vi "main.vi"() -> ()   [LabVIEW 2024]
uses:
  Controller/Controller/Controller.lvclass
  Applications/National Instruments/LabVIEW 2024 64-bit/vi.lib/ActorFramework/Actor/Actor.lvclass
  <vilib>/ActorFramework/Message Enqueuer/Message Enqueuer.lvclass/Message Enqueuer.ctl
  <vilib>/ActorFramework/Message Enqueuer/Enqueue.vi
  Controller/Controller Messages/Reset Contestant Lights Msg/Reset Contestant Lights Msg.lvclass
  Applications/National Instruments/LabVIEW 2024 64-bit/vi.lib/ActorFramework/Message/Message.lvclass
  <vilib>/ActorFramework/Stop Msg/Stop Msg.lvclass
  Controller/Controller Messages/Welcome Animation Msg/Welcome Animation Msg.lvclass
  <vilib>/ActorFramework/Message Priority Queue/Priority Enqueue.vi
  <vilib>/ActorFramework/Actor/Actor.lvclass
panel:
  in  "Hype":bool
  in  "Stop Button":bool
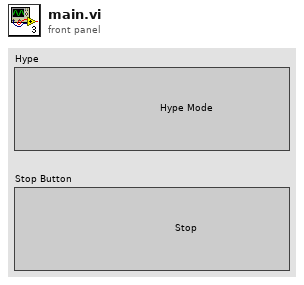
[diagram p1: front panel]
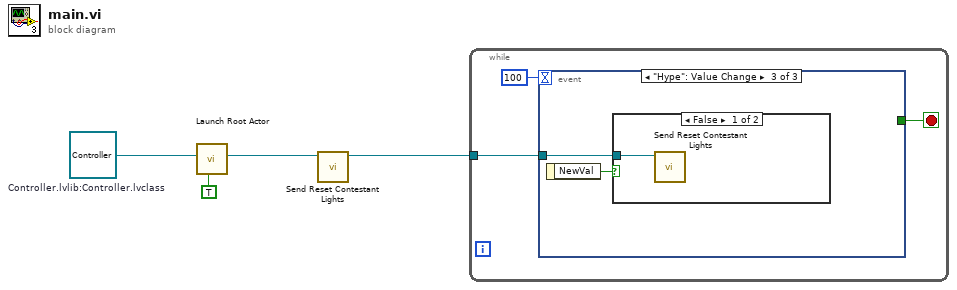
[diagram p0: block diagram]
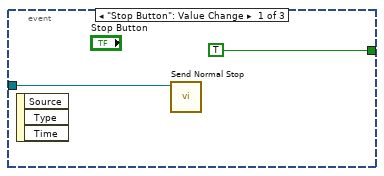
[diagram p2: hidden frame]
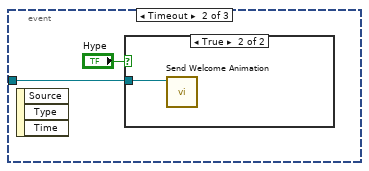
[diagram p3: hidden frame]
diagram:
  w4 = refnum<class "Controller.lvclass"> refnum  # Controller.lvlib:Controller.lvclass
  n1 = call <vilib>:"Launch Root Actor.vi"("Open Actor Core front panel? (F)"=TRUE, "Actor"=w4) -> ("Actor's Enqueuer"=w2:refnum<class "Message Enqueuer.lvclass">)  [unwired: 8 in, 1 out]
  n2 = call "Send Reset Contestant Lights.vi"("Message Enqueuer"=w2) -> ("Message Enqueuer out"=w1:refnum<class "Message Enqueuer.lvclass">)  [unwired: 9 in, 1 out]
  n3 = while {
    tunnel: w1 -> [w6]
    stop <- w7 stop-if-true
    n4 = event shown="[2] \"Hype\": Value Change" {
      selector: _ -> [_ _ _]
      dyn-events: _ -> [_ _ _]
      timeout: 100 -> [_ _ _]
      tunnel: [TRUE ("Stop Button") _ _] -> w7
      tunnel: w6 -> [w8 w10 w13]
      event "Stop Button": Value Change {
        n5 = event-data() -> ()  [unwired: 1 in, 3 out]
        n6 = call <vilib>:"Send Normal Stop.vi"("Message Enqueuer"=w8) -> ()  [unwired: 10 in, 1 out]
      }
      event Timeout {
        n7 = event-data() -> ()  [unwired: 1 in, 3 out]
        n8 = case shown="True" "Hype" {
          tunnel: w10 -> [_ w12]
          frame False {
          }
          frame True {
            n9 = call "Send Welcome Animation.vi"("Message Enqueuer"=w12) -> ()  [unwired: 9 in, 2 out]
          }
        }
      }
      event "Hype": Value Change {
        n10 = event-data() -> ("NewVal"=w14:bool)  [unwired: 1 in]
        n11 = case shown="False" w14 {
          tunnel: w13 -> [w15 _]
          frame False {
            n12 = call "Send Reset Contestant Lights.vi"("Message Enqueuer"=w15) -> ()  [unwired: 9 in, 2 out]
          }
          frame True {
          }
        }
      }
    }
  }
